vi "DBTester3.vi"() -> ()   [LabVIEW 2015]
uses:
  BERTTA.dll
panel:
  out "save data":dbl
  out "Mettler":dynamicdata(graph)
  in  "Device port":i32=6
  out "Weight":dbl
  out "Weight 2":dbl
  in  "Device port 2":i32=2
  out "rc":i32
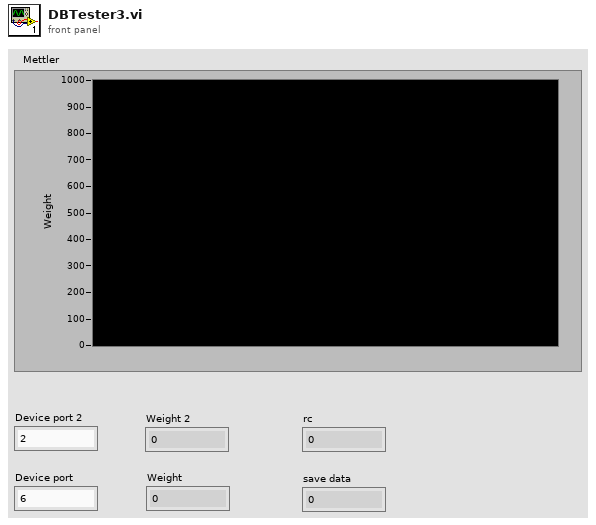
[diagram p1: front panel]
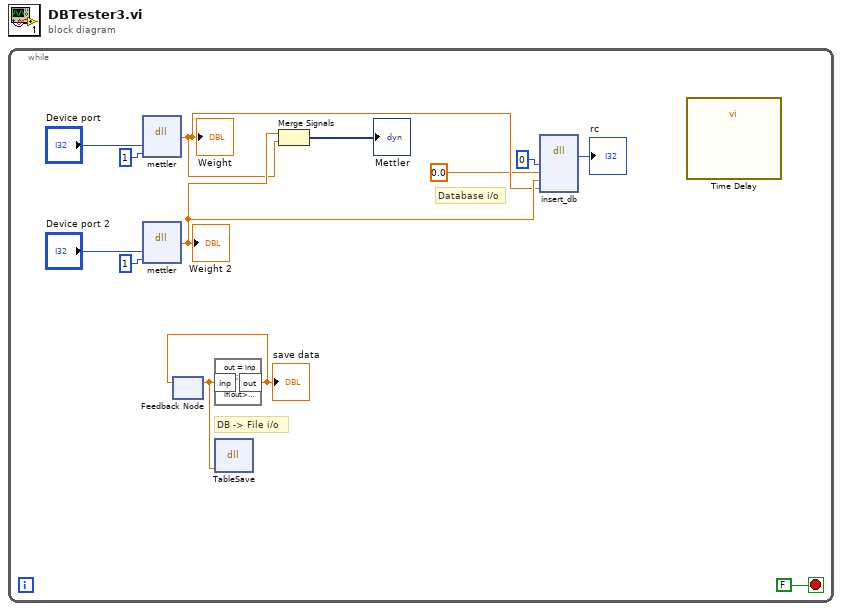
[diagram p0: block diagram]
diagram:
  n1 = while {
    stop <- FALSE stop-if-true
    # "DB -> File i/o"
    # "Database i/o"
    n2 = dll-call lib="C:/Users/xlaraser/Documents/Visual Studio 2017/Projects/Bertta/BERTTA/Debug/BERTTA.dll" fn="mettler"("port"="Device port", "msg"=1) -> ("return type"=w6:dbl)  [unwired: 5 in, 2 out]
    "Weight" <- w6
    n3 = dll-call lib="C:/Users/xlaraser/Documents/Visual Studio 2017/Projects/Bertta/BERTTA/Debug/BERTTA.dll" fn="mettler"("port"="Device port 2", "msg"=1) -> ("return type"=w7:dbl)  [unwired: 5 in, 2 out]
    "Weight 2" <- w7
    n4 = feedback #1() -> (w2:dbl)  [unwired: 1 in]
    n5 = formula code="out = inp + 1;\n\nif(out>5) out = 0;"("inp"=w2) -> ("out"=w1:dbl)
    "save data" <- w1
    n6 = feedback-in #1(w1) -> ()
    n7 = dll-call lib="C:/Users/xlaraser/Documents/Visual Studio 2017/Projects/Bertta/BERTTA/Debug/BERTTA.dll" fn="TableSave"("exec"=w2) -> ()  [unwired: 5 in, 2 out]
    n8 = Merge Signals(w7, w6) -> (→"Mettler":dynamicdata)
    n9 = dll-call lib="C:/Users/xlaraser/Documents/Visual Studio 2017/Projects/Bertta/BERTTA/Debug/BERTTA.dll" fn="insert_db"("heidolph"=0, "lauda"=0.0, "mettler1"=w7, "mettler2"=w6) -> ("return type"=→"rc":i32)  [unwired: 7 in, 2 out]
    n10 = call "Time Delay"() -> ()  [unwired: 11 in, 1 out]
  }
